vi "MultiGrid_v3.vi"() -> ()   [LabVIEW 2014]
uses:
  <userlib>/Nanonis Prog Interface V5/Scan/Grid/GridPatternGet.vi
  <userlib>/Nanonis Prog Interface V5/Nanonis Prog Interface.lvlib
panel:
  in  "take Image 2x":bool
  out "External VI path":path
  in  "done Setting":bool=TRUE
  in  "Get Frame&Grid":bool
  in  "index (row)":i32=3
  in  "GO":bool
  out "Y offset":dbl format="%#_6p"
  out "X offset":dbl format="%#_6p"
  in  "Grid":i32(listbox)=3
  in  "Frame":i32(listbox)=3
  in  "Cloud Grid":bool
  in  "GridSettings":T1={"Imaging Current"=5e-11, "STS Current"=1e-09, "Start value (V)"=-0.05, "End value (V)"=0.05, "Number of points (0=no change)"=256, "File name"="single_mol_shortSTS", "DC pixel"=64.0, "Grid X"=0.0, "Grid Y"=0.0, "Sweeps"=8.0}
  in  "Polling (s)":u32=600
  out "Status":string
  out "#Grids":i32=2
  in  "MultiGrid":i32(listbox)=2
  # "0 for no change"
  # "Stop the Nanoishelper, Run labbook helper"
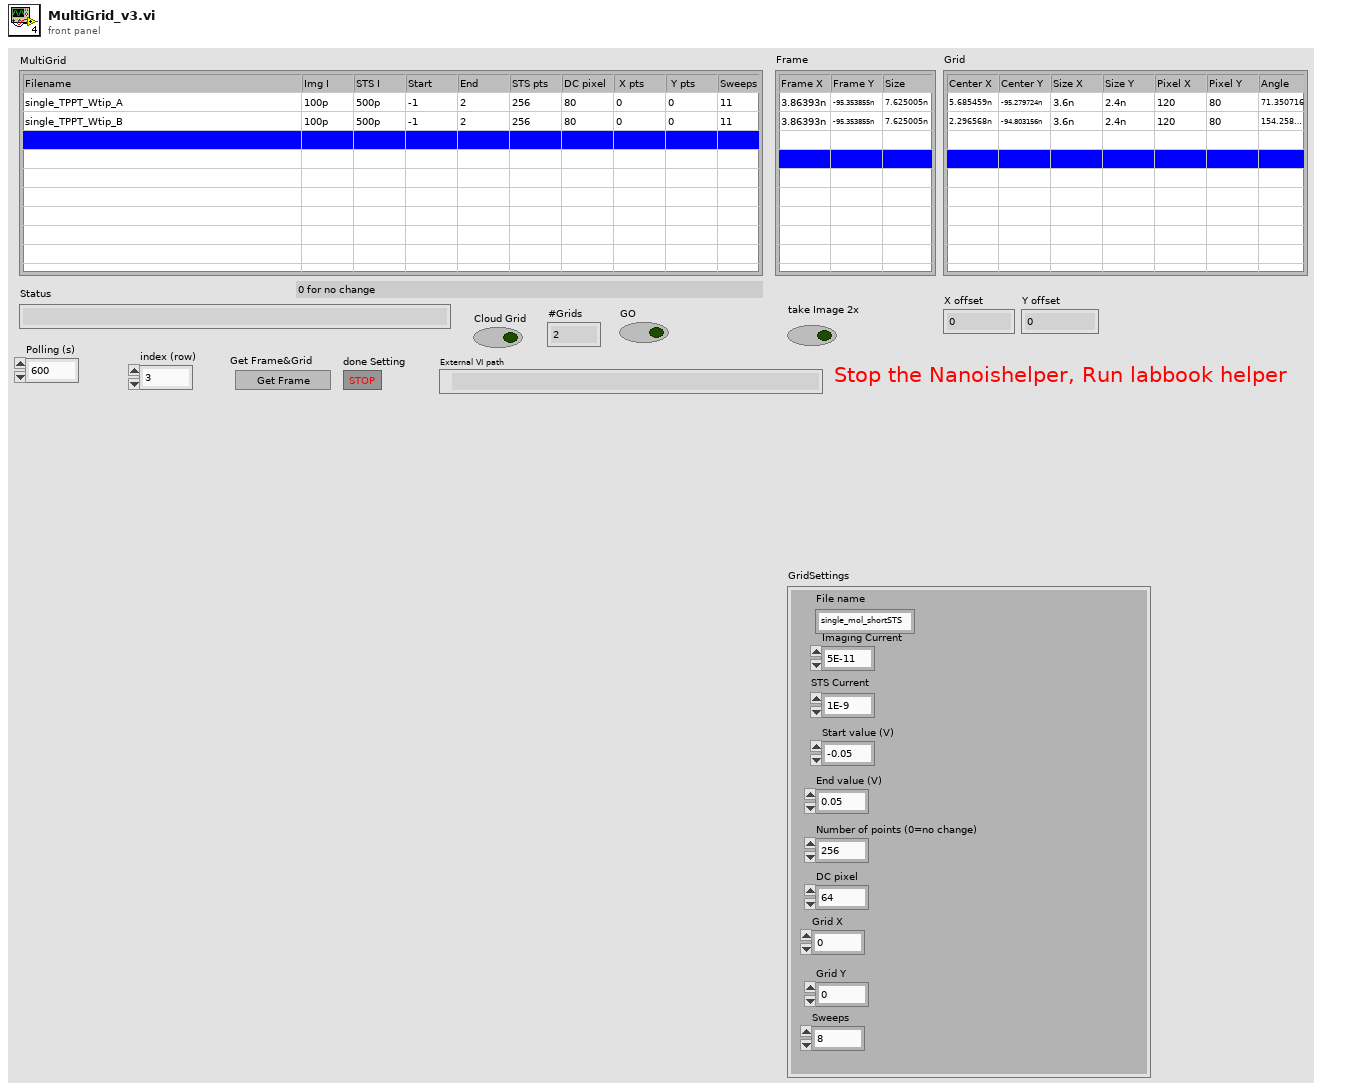
[diagram p1: front panel]
types:
  T1 = cluster{"Imaging Current":sgl, "STS Current":sgl, "Start value (V)":sgl, "End value (V)":sgl, "Number of points (0=no change)":i32, "File name":string, "DC pixel":dbl, "Grid X":dbl, "Grid Y":dbl, "Sweeps":dbl}
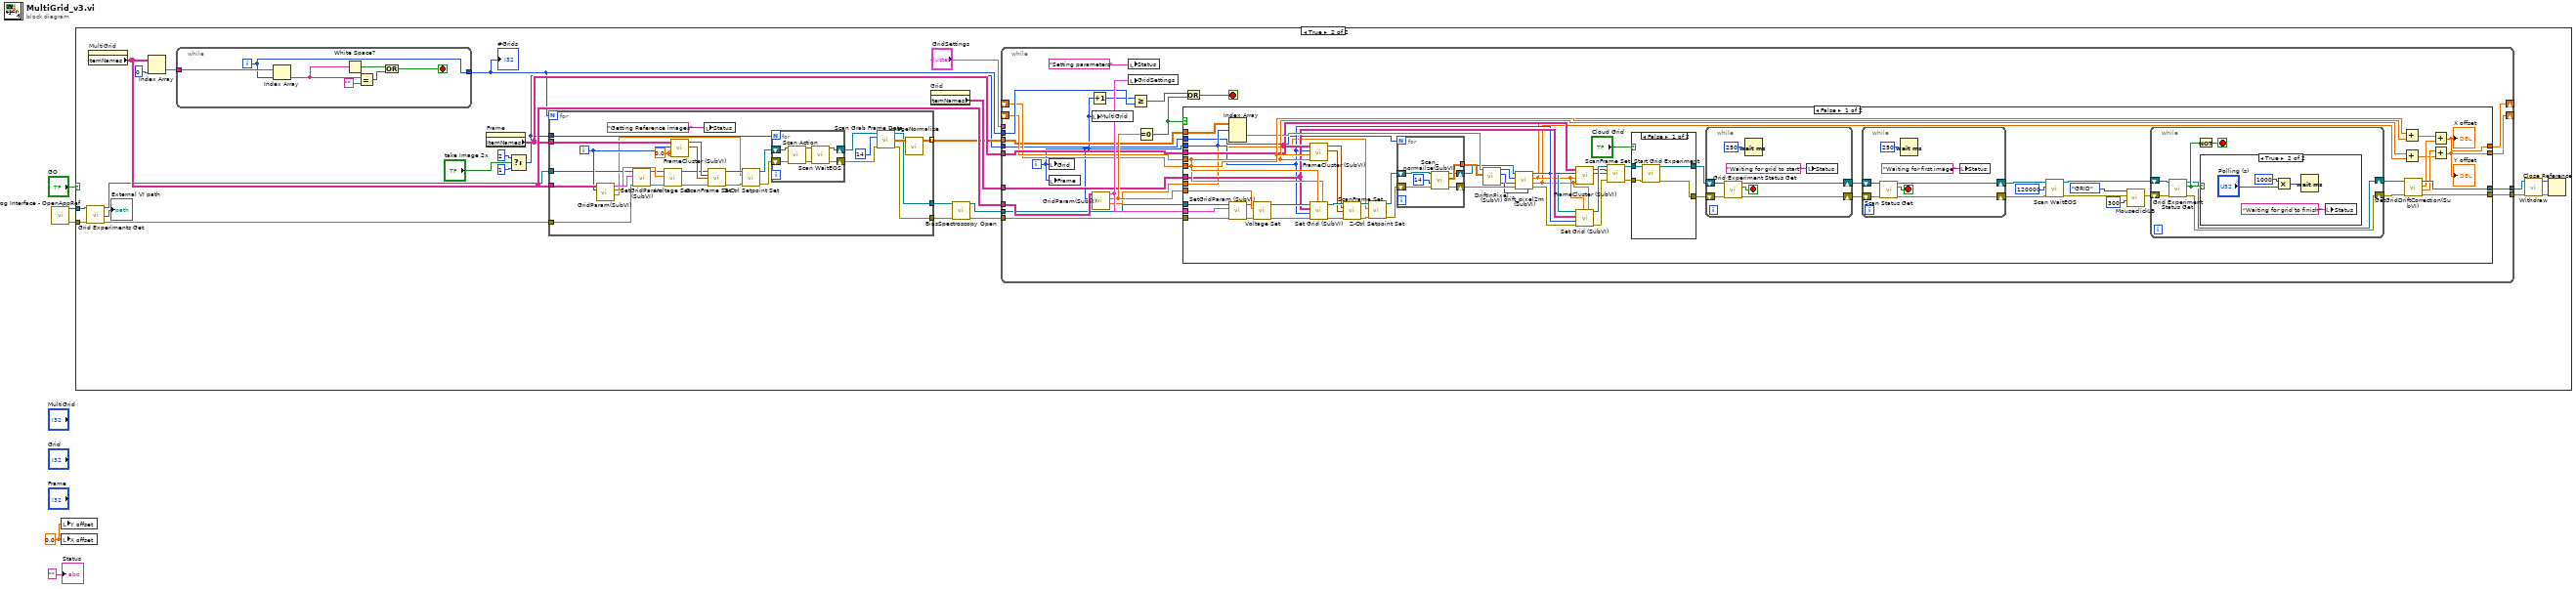
[diagram p0: block diagram]
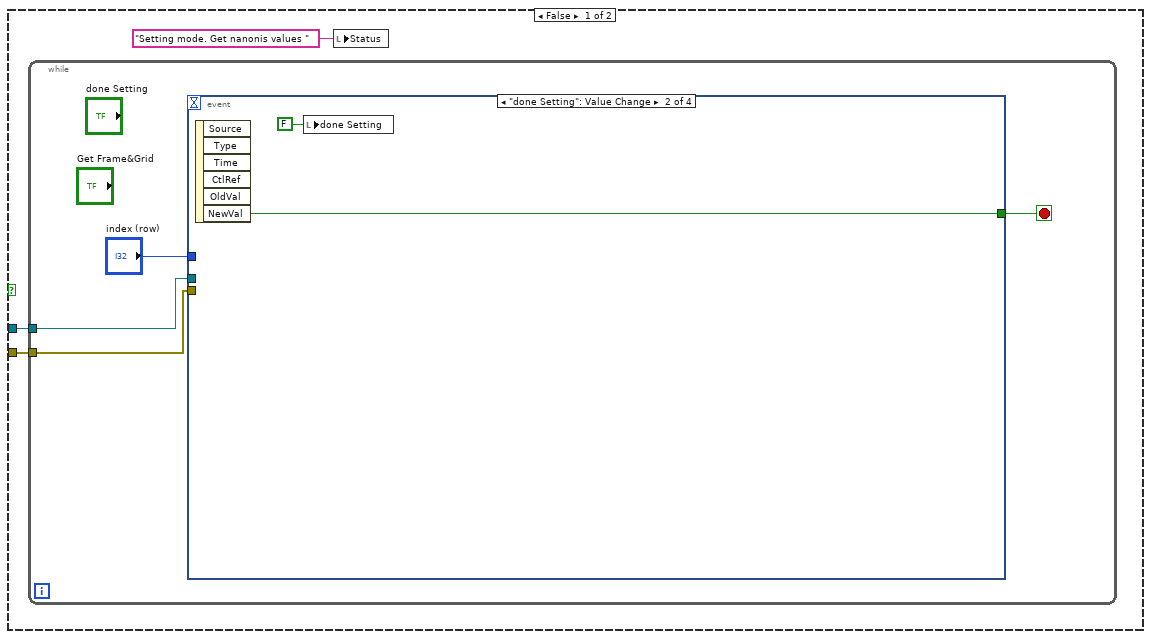
[diagram p2: hidden frame]
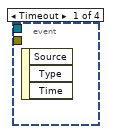
[diagram p3: hidden frame]
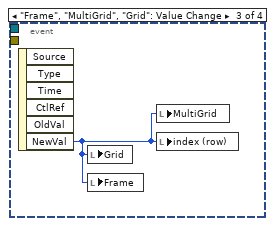
[diagram p4: hidden frame]
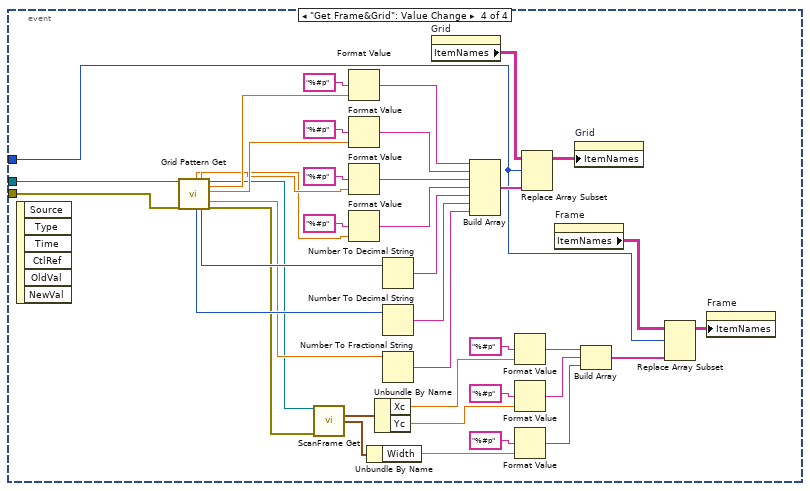
[diagram p5: hidden frame]
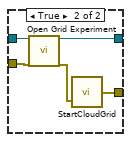
[diagram p6: hidden frame]
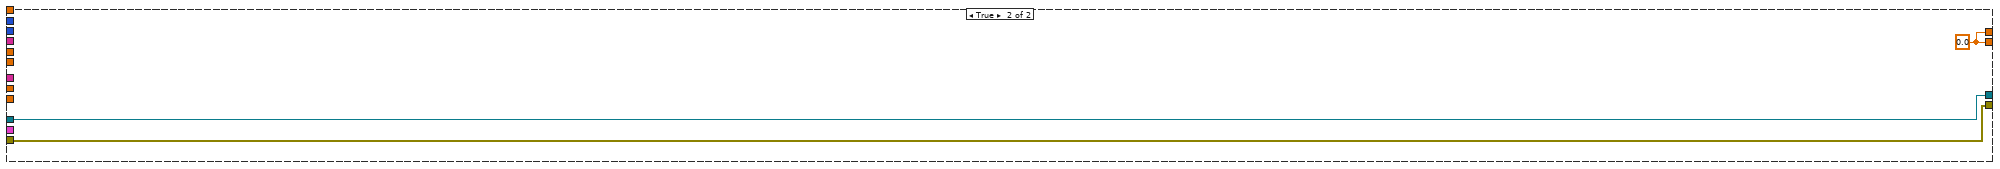
[diagram p8: hidden frame]
diagram:
  w4 = 0.0 ("Y offset")
  n1 = call <userlib>:"Prog Interface - OpenAppRef.vi"() -> ("Error out"=w1:errorcluster, "Application reference"=w2:refnum<vi>)  [unwired: 6 in]
  n2 = local write "Y offset"(w4) -> ()
  n3 = local write "X offset"(w4) -> ()
  n4 = case shown="True" "GO" {
    tunnel: w2 -> [w8 w64]
    tunnel: w1 -> [w7 w61]
    frame False {
      n5 = while {
        tunnel: w8 -> [w11]
        tunnel: w7 -> [w10]
        stop <- w9 stop-if-true
        n6 = event shown="[1] \"done Setting\": Value Change" {
          selector: _ -> [_ _ _ _]
          dyn-events: _ -> [_ _ _ _]
          timeout: _ -> [_ _ _ _]
          tunnel: "index (row)" -> [_ _ _ w32]
          tunnel: w11 -> [_ _ _ w24]
          tunnel: w10 -> [_ _ _ w23]
          tunnel: [_ w14 _ _] -> w9
          event Timeout {
            n7 = event-data() -> ()  [unwired: 1 in, 3 out]
          }
          event "done Setting": Value Change {
            n8 = event-data() -> ("NewVal"=w14:bool)  [unwired: 1 in, 5 out]
            n9 = local write "done Setting"(FALSE ("done Setting")) -> ()
          }
          event "Frame", "MultiGrid", "Grid": Value Change {
            n10 = event-data() -> ("NewVal"=w15:i32)  [unwired: 1 in, 5 out]
            n11 = local write "Grid"(w15) -> ()
            n12 = local write "Frame"(w15) -> ()
            n13 = local write "MultiGrid"(w15) -> ()
            n14 = local write "index (row)"(w15) -> ()
          }
          event "Get Frame&Grid": Value Change {
            n15 = event-data() -> ()  [unwired: 1 in, 6 out]
            n16 = call-poly <userlib>:"Grid Pattern Get.vi"("Application ref in"=w24, "error in (no error)"=w23) -> ("Height (m)"=w43:sgl, "Points Y"=w38:i32, "Width (m)"=w46:sgl, "Points X"=w40:i32, "Application ref out"=w22:refnum<vi>, "Center Xc (m)"=w52:sgl, "Center Yc (m)"=w48:sgl, "Angle (°)"=w36:sgl, "error out"=w21:errorcluster)  [unwired: 9 in]
            n17 = call <userlib>:"ScanFrame Get.vi"("Application ref in"=w22, "error in (no error)"=w21) -> ("Center coordinates (m)"=w19:cluster{"Xc":sgl, "Yc":sgl}, "Size (m)"=w20:cluster{"Width":sgl, "Height":sgl})  [unwired: 9 in, 3 out]
            n18 = Format Value(format string="%#p", value (0)=w52) -> (output string=w51:string)  [unwired: 1 in]
            n19 = Format Value(format string="%#p", value (0)=w48) -> (output string=w47:string)  [unwired: 1 in]
            n20 = Format Value(format string="%#p", value (0)=w46) -> (output string=w44:string)  [unwired: 1 in]
            n21 = Format Value(format string="%#p", value (0)=w43) -> (output string=w41:string)  [unwired: 1 in]
            n22 = Unbundle By Name(w20) -> ("Width"=w16:sgl)
            n23 = Unbundle By Name(w19) -> ("Xc"=w18:sgl, "Yc"=w17:sgl)
            n24 = Number To Decimal String(number=w40) -> (decimal integer string=w39:string)  [unwired: 1 in]
            n25 = Number To Decimal String(number=w38) -> (decimal integer string=w37:string)  [unwired: 1 in]
            n26 = Number To Fractional String(number=w36) -> (F-format string=w35:string)  [unwired: 3 in]
            n27 = property on="Grid" class="MCListbox (strict)"() -> ("ItemNames"=w55:string[][])  [unwired: 2 in, 2 out]
            n28 = Build Array(w51, w47, w44, w41, w39, w37, w35) -> (w54:string[])
            n29 = Format Value(format string="%#p", value (0)=w18) -> (output string=w28:string)  [unwired: 1 in]
            n30 = Format Value(format string="%#p", value (0)=w17) -> (output string=w27:string)  [unwired: 1 in]
            n31 = Format Value(format string="%#p", value (0)=w16) -> (output string=w26:string)  [unwired: 1 in]
            n32 = Replace Array Subset(array=w55, new element=w54, index (row)=w32) -> (w50:string[][])  [unwired: 1 in]
            n33 = property on="Frame" class="MCListbox (strict)"() -> ("ItemNames"=w34:string[][])  [unwired: 2 in, 2 out]
            n34 = property on="Grid" class="MCListbox (strict)"("ItemNames"=w50) -> ()  [unwired: 2 in, 2 out]
            n35 = Build Array(w28, w27, w26) -> (w25:string[])
            n36 = Replace Array Subset(array=w34, new element=w25, index (row)=w32) -> (w33:string[][])  [unwired: 1 in]
            n37 = property on="Frame" class="MCListbox (strict)"("ItemNames"=w33) -> ()  [unwired: 2 in, 2 out]
          }
        }
      }
      n38 = local write "Status"("Setting mode. Get nanonis values " ("Status")) -> ()
    }
    frame True {
      n39 = call <userlib>:"Grid Experiments Get.vi"("Application ref in"=w64, "error in (no error)"=w61) -> ("Application ref out"=w63:refnum<vi>, "External VI path"=→"External VI path":path, "error out"=w62:errorcluster)  [unwired: 11 in, 4 out]
      n40 = property on="MultiGrid" class="MCListbox (strict)"() -> ("ItemNames"=w70:string[][])  [unwired: 2 in, 2 out]
      n41 = Index Array(array=w70, index (col)=0 ("disabled index (col)")) -> (element=w77:string[])  [unwired: 1 in]
      n42 = while {
        tunnel: w77 -> [w250]
        tunnel: [w244] -> w66
        i -> [w244]
        stop <- w246 stop-if-true
        n43 = Index Array(array=w250, index=w244) -> (element=w249:string)
        n44 = White Space?(1:w249) -> (0:w247:bool)
        n45 = Equal?(x=w249, y="") -> (x = y?=w245:bool)
        n46 = Or(x=w247, y=w245) -> (x .or. y?=w246:bool)
      }
      "#Grids" <- w66
      n47 = property on="Frame" class="MCListbox (strict)"() -> ("ItemNames"=w69:string[][])  [unwired: 2 in, 2 out]
      n48 = Select(t=2, s="take Image 2x", f=1) -> (s? t:f=w56:i32)
      n49 = for {
        N: w66 -> [_]
        tunnel: w70 -> [w106]
        tunnel: w69 -> [w103]
        tunnel: w63 -> [w98]
        tunnel: w62 -> [w97]
        tunnel: [w90] -> w68
        tunnel: [w89] -> w67
        tunnel: [w87] -> w65 mode=indexing
        tunnel: w56 -> [w81]
        i -> [w101]
        w102 = 0.0 ("x offset")
        n50 = call "GridParam(SubVI).vi"("Numeric in"=w101, "ItemNames"=w106) -> ("Img Current"=w82:dbl, "Bias"=w104:dbl, "GridSettings"=w105:T1)  [unwired: 7 in]
        n51 = call "SetGridParam (SubVI).vi"("error in (no error)"=w97, "GridSettings"=w105, "Application in"=w98) -> ("Error out"=w96:errorcluster, "Application ref out"=w95:refnum<vi>)  [unwired: 7 in]
        n52 = call <userlib>:"Voltage Set.vi"("Error in (no error)"=w96, "Bias (V)"=w104, "Application ref in"=w95) -> ("Error out"=w93:errorcluster, "Application ref out"=w94:refnum<vi>)  [unwired: 7 in]
        n53 = call "FrameCluster (SubVI).vi"("y offset"=w102, "x offset"=w102, "index (row)"=w101, "ItemNames"=w103) -> ("Size (m)"=w100:cluster{"Width":sgl, "Height":sgl}, "Center coordinates (m)"=w99:cluster{"Xc":sgl, "Yc":sgl})  [unwired: 6 in]
        n54 = local write "Status"("Getting Reference images" ("Status")) -> ()
        n55 = call <userlib>:"ScanFrame Set.vi"("Application ref in"=w94, "Center coordinates (m)"=w99, "Size (m)"=w100, "error in (no error)"=w93) -> ("Application ref out"=w86:refnum<vi>, "error out"=w85:errorcluster)  [unwired: 10 in]
        n56 = call <userlib>:"Z-Ctrl Setpoint Set.vi"("error in (no error)"=w85, "Z Controller setpoint"=w82, "Application ref in"=w86) -> ("error out"=w83:errorcluster, "Application ref out"=w84:refnum<vi>)  [unwired: 7 in]
        n57 = for {
          N: w81 -> [_]
          shift-right: [w113] -> w108
          shift-left: w84 -> [w110]
          shift-right: [w111] -> w92
          shift-left: w83 -> [w109]
          n58 = call <userlib>:"Scan Action.vi"("error in (no error)"=w109, "Application ref in"=w110) -> ("error out"=w112:errorcluster, "Application ref out"=w114:refnum<vi>)  [unwired: 7 in]
          n59 = call <userlib>:"Scan WaitEOS.vi"("error in (no error)"=w112, "Application ref in"=w114) -> ("error out"=w111:errorcluster, "Application ref out"=w113:refnum<vi>)  [unwired: 5 in, 2 out]
        }
        n60 = call <userlib>:"Scan Grab Frame Data.vi"("Application ref in"=w108, "Channel index (0-23)"=u8 14, "error in (no error)"=w92) -> ("Application ref out"=w90:refnum<vi>, "Scan frame data"=w107:sgl[][], "error out"=w89:errorcluster)  [unwired: 8 in, 2 out]
        n61 = call "imageNormalize.vi"("Data"=w107) -> ("Array"=w87:dbl[][])  [unwired: 10 in]
      }
      n62 = property on="Grid" class="MCListbox (strict)"() -> ("ItemNames"=w71:string[][])  [unwired: 2 in, 2 out]
      n63 = call <userlib>:"BiasSpectroscopy Open.vi"("Application ref in"=w68, "Error in (no error)"=w67) -> ("Application ref out"=w73:refnum<vi>, "Error out"=w72:errorcluster)  [unwired: 12 in]
      n64 = while {
        tunnel: w70 -> [w137]
        tunnel: w73 -> [w131]
        tunnel: w72 -> [w130]
        tunnel: "GridSettings" -> [_]
        tunnel: [w129] -> w80
        tunnel: [w132] -> w79
        tunnel: w66 -> [w133]
        shift-right: [w124] -> _
        shift-left: _ -> [w119]
        shift-right: [w123] -> _
        shift-left: _ -> [w120]
        tunnel: w71 -> [w122]
        tunnel: w69 -> [w121]
        tunnel: w65 -> [w118]
        tunnel: w56 -> [w115]
        i -> [w116]
        stop <- w128 stop-if-true
        n65 = local write "Grid"(w116) -> ()
        n66 = local write "Frame"(w116) -> ()
        n67 = Increment(x=w116) -> (x+1=w127:i32)
        n68 = local write "MultiGrid"(w116) -> ()
        n69 = call "GridParam(SubVI).vi"("Numeric in"=w116, "ItemNames"=w137) -> ("Img Current"=w117:dbl, "Bias"=w125:dbl, "GridSettings"=w136:T1)  [unwired: 7 in]
        n70 = local write "Status"("Setting parameters" ("Status")) -> ()
        n71 = local write "GridSettings"(w136) -> ()
        n72 = Greater Or Equal?(x=w127, y=w133) -> (x >= y?=w134:bool)
        n73 = Equal To 0?(x=w125) -> (x = 0?=w126:bool)
        n74 = case shown="False" w126 {
          tunnel: w136 -> [w201 _]
          tunnel: [w179 w242] -> w132
          tunnel: w131 -> [w200 w243]
          tunnel: w130 -> [w199 w242]
          tunnel: [w181 w243] -> w129
          tunnel: w125 -> [w185 _]
          tunnel: [w169 w241] -> w124
          tunnel: [w170 w241] -> w123
          tunnel: w122 -> [w153 _]
          tunnel: w116 -> [w152 _]
          tunnel: w121 -> [w154 _]
          tunnel: w120 -> [w167 _]
          tunnel: w119 -> [w168 _]
          tunnel: w118 -> [w161 _]
          tunnel: w117 -> [w139 _]
          tunnel: w115 -> [w138 _]
          frame False {
            n75 = Index Array(array=w161, index (dim 0)=w152) -> (element=w160:dbl[][])  [unwired: 2 in]
            n76 = call "SetGridParam (SubVI).vi"("error in (no error)"=w199, "GridSettings"=w201, "Application in"=w200) -> ("Error out"=w183:errorcluster, "Application ref out"=w184:refnum<vi>)  [unwired: 7 in]
            n77 = call <userlib>:"Voltage Set.vi"("Error in (no error)"=w183, "Bias (V)"=w185, "Application ref in"=w184) -> ("Error out"=w171:errorcluster, "Application ref out"=w176:refnum<vi>)  [unwired: 7 in]
            n78 = call "FrameCluster (SubVI).vi"("y offset"=w167, "x offset"=w168, "index (row)"=w152, "ItemNames"=w154) -> ("Size (m)"=w173:cluster{"Width":sgl, "Height":sgl}, "Center coordinates (m)"=w174:cluster{"Xc":sgl, "Yc":sgl})  [unwired: 6 in]
            n79 = call "Set Grid (SubVI).vi"("y offset"=w167, "x offset"=w168, "error in (no error)"=w171, "index (row)"=w152, "ItemNames"=w153, "Application in"=w176) -> ("error out"=w172:errorcluster, "Application out"=w175:refnum<vi>)  [unwired: 4 in]
            n80 = call <userlib>:"ScanFrame Set.vi"("Application ref in"=w175, "Center coordinates (m)"=w174, "Size (m)"=w173, "error in (no error)"=w172) -> ("Application ref out"=w166:refnum<vi>, "error out"=w165:errorcluster)  [unwired: 10 in]
            n81 = call <userlib>:"Z-Ctrl Setpoint Set.vi"("error in (no error)"=w165, "Z Controller setpoint"=w139, "Application ref in"=w166) -> ("error out"=w163:errorcluster, "Application ref out"=w164:refnum<vi>)  [unwired: 7 in]
            n82 = for {
              N: w138 -> [_]
              tunnel: [w204] -> w162
              shift-right: [w203] -> w159
              shift-left: w164 -> [w207]
              shift-right: [w202] -> w158
              shift-left: w163 -> [w206]
              n83 = call "Scan_normailze(SubVI).vi"("error in (no error)"=w206, "Channel index (0-23)"=u8 14, "Application in"=w207) -> ("error out"=w202:errorcluster, "Array"=w204:dbl[][], "Application out"=w203:refnum<vi>)  [unwired: 6 in]
            }
            n84 = call "DriftInPixel (SubVI).vi"("New image"=w162, "Ref image"=w160) -> ("pixel"=w157:i32, "Y drift"=w155:i32, "X drift"=w156:i32)  [unwired: 7 in]
            n85 = call "drift_pixel2m (SubVI).vi"("Application in"=w159, "X drift"=w156, "Y drift"=w155, "error in"=w158, "Drift correction Pixels"=w157) -> ("Application out"=w151:refnum<vi>, "x drift"=w141:sgl, "y drift"=w140:sgl, "error out"=w150:errorcluster)  [unwired: 1 in]
            n86 = call "FrameCluster (SubVI).vi"("y offset"=w140, "x offset"=w141, "index (row)"=w152, "ItemNames"=w154) -> ("Size (m)"=w146:cluster{"Width":sgl, "Height":sgl}, "Center coordinates (m)"=w147:cluster{"Xc":sgl, "Yc":sgl})  [unwired: 6 in]
            n87 = call "Set Grid (SubVI).vi"("y offset"=w140, "x offset"=w141, "error in (no error)"=w150, "index (row)"=w152, "ItemNames"=w153, "Application in"=w151) -> ("error out"=w149:errorcluster, "Application out"=w148:refnum<vi>)  [unwired: 4 in]
            n88 = call <userlib>:"ScanFrame Set.vi"("Application ref in"=w148, "Center coordinates (m)"=w147, "Size (m)"=w146, "error in (no error)"=w149) -> ("Application ref out"=w145:refnum<vi>, "error out"=w144:errorcluster)  [unwired: 10 in]
            n89 = case shown="False" "Cloud Grid" {
              tunnel: w144 -> [w225 w228]
              tunnel: [w224 w229] -> w197
              tunnel: [w223 w227] -> w196
              tunnel: w145 -> [w222 w230]
              frame False {
                n90 = call <userlib>:"Start Grid Experiment.vi"("Application ref in"=w222, "error in (no error)"=w225) -> ("Application ref out"=w224:refnum<vi>, "error out"=w223:errorcluster)  [unwired: 16 in]
              }
              frame True {
                n91 = call <userlib>:"Open Grid Experiment.vi"("Application ref in"=w230, "error in (no error)"=w228) -> ("Application ref out"=w229:refnum<vi>, "error out"=w226:errorcluster)  [unwired: 16 in]
                n92 = call "StartCloudGrid.vi"("error in (no error)"=w226) -> ("error out"=w227:errorcluster)  [unwired: 1 in]
              }
            }
            n93 = while {
              shift-right: [w221] -> w190
              shift-left: w197 -> [w217]
              shift-right: [w216] -> w186
              shift-left: w196 -> [w220]
              stop <- w215 stop-if-true
              n94 = call <userlib>:"Grid Experiment Status Get.vi"("error in (no error)"=w220, "Application ref in"=w217) -> ("error out"=w216:errorcluster, "Running?"=w215:bool, "Application ref out"=w221:refnum<vi>)  [unwired: 7 in]
              n95 = Wait (ms)(milliseconds to wait=u32 250) -> ()  [unwired: 1 out]
              n96 = local write "Status"("Waiting for grid to start" ("Status")) -> ()
            }
            n97 = while {
              shift-right: [w212] -> w189
              shift-left: w190 -> [w213]
              shift-right: [w211] -> w188
              shift-left: w186 -> [w214]
              stop <- w210 stop-if-true
              n98 = call <userlib>:"Scan Status Get.vi"("error in (no error)"=w214, "Application ref in"=w213) -> ("error out"=w211:errorcluster, "Scanning?"=w210:bool, "Application ref out"=w212:refnum<vi>)  [unwired: 6 in]
              n99 = Wait (ms)(milliseconds to wait=u32 250) -> ()  [unwired: 1 out]
              n100 = local write "Status"("Waiting for first image" ("Status")) -> ()
            }
            n101 = call <userlib>:"Scan WaitEOS.vi"("error in (no error)"=w188, "Timeout in ms (-1)"=120000, "Application ref in"=w189) -> ("error out"=w192:errorcluster, "Application ref out"=w191:refnum<vi>)  [unwired: 4 in, 2 out]
            n102 = call "MouseclickLB.vi"("nMilliseconds"=300, "error in (no error)"=w192, "Click"=enum16{"Header", "TOPO", "STS", "GRID"}."GRID") -> ("error out"=w195:errorcluster)  [unwired: 8 in]
            n103 = while {
              shift-right: [w233] -> w182
              shift-left: w191 -> [w234]
              shift-right: [w231] -> w180
              shift-left: w195 -> [w232]
              stop <- w236 stop-if-true
              n104 = call <userlib>:"Grid Experiment Status Get.vi"("error in (no error)"=w232, "Application ref in"=w234) -> ("error out"=w231:errorcluster, "Running?"=w235:bool, "Application ref out"=w233:refnum<vi>)  [unwired: 7 in]
              n105 = Not(x=w235) -> (.not. x?=w236:bool)
              n106 = case shown="True" w235 {
                frame False {
                }
                frame True {
                  n107 = Multiply(x=u32 1000, y="Polling (s)") -> (x*y=w239:u32)
                  n108 = Wait (ms)(milliseconds to wait=w239) -> ()  [unwired: 1 out]
                  n109 = local write "Status"("Waiting for grid to finish" ("Status")) -> ()
                }
              }
            }
            n110 = Add(x=w141, y=w168) -> (x+y=w143:dbl)
            n111 = Add(x=w167, y=w140) -> (x+y=w142:dbl)
            n112 = call "GetGridDriftCorrection(SubVI).vi"("error in (no error)"=w180, "Application in"=w182) -> ("Error out"=w179:errorcluster, "Y offset"=w177:dbl, "X offset"=w178:dbl, "Application ref out"=w181:refnum<vi>)  [unwired: 6 in]
            n113 = Add(x=w143, y=w178) -> (x+y=w169:dbl)
            "X offset" <- w169
            n114 = Add(x=w177, y=w142) -> (x+y=w170:dbl)
            "Y offset" <- w170
          }
          frame True {
            w241 = 0.0 ("X offset")
          }
        }
        n115 = Or(x=w134, y=w126) -> (x .or. y?=w128:bool)
      }
      n116 = call <userlib>:"Withdraw.vi"("Error in (no error)"=w79, "Application ref in"=w80) -> ("Error out"=w74:errorcluster, "Application ref out"=w75:refnum<vi>)  [unwired: 8 in]
      n117 = Close Reference(reference=w75, error in (no error)=w74) -> ()  [unwired: 1 out]
    }
  }
  "Status" <- "" ("Status")
